vi "TCP Error Handler.vi"(3 "Error In":errorcluster, 4 "Info":string) -> (0 "Error Out":errorcluster, 1 "Info":string, 2 "TCP":bool)   [LabVIEW 2018]
doc: "Also checks for R&D FW or DAS FW"
uses:
  Type Defs/RT Command.ctl
  Type Defs/Global Action.ctl
  GC-MSMSDevlopment/Configuration/_Global Configuration.vi
  <vilib>/Utility/error.llb/Error Cluster From Error Code.vi
  <vilib>/ErrorRing/Error Ring.xnode
panel:
  # "All TCP/IP Errors are handle by this methode"
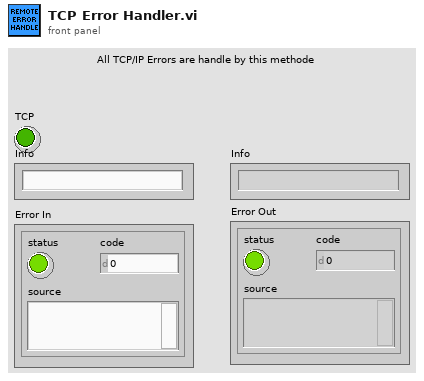
[diagram p1: front panel]
types:
  T1 = typedef "RT Command.ctl" = enum16{"xml Start Run", "xml Start Actual Run", "xml Stop Run", "xml Runtime Update", "xml Get Status", "xml Get Table", "xml Set Table", "xml Get Configuration", "xml System Status", "xml Set LC Input Logic", "xml Get Data", "xml Get Info", "Start", "StartActualRun", "Stop", "Runtime Update", "Get Data", "Get Info", "Get Status", "Get Param", "Get Config", "Get Table", "Read ADC", "Set Oscillator", "Update Config", "Update Table", "Set All Pol", "Set Pol and DC", "Set Max Mass", "Toggle RP", "Toggle EL", "Set PIC", "Initialize Turbo", "Send Turbo Comm", "Close Turbo", "P1", "P2", "P3", "Send Serial", "Set LC Out", "Get LC In", "Read VAC", "Test Table", "Toggle Power", "Get Startup", "Set Startup", "Get ADC Table", "Set ADC Table", "Get Brief Status", "Get Detail Status", "Auxiliary Update", "Set CC Logics", "Set CC Input Logics", "Ignore Error", "invalid"}
  T2 = typedef "Global Action.ctl" = enum16{"Write", "Read"}
  T3 = typedef "Global Configrations.ctl" = cluster{"Model Name":enum16{"QSight 110", "QSight 120", "QSight 210", "QSight 220", "QSight 410", "QSight 420", "IONICS 3Q 110", "IONICS 3Q 120", "IONICS 3Q 210", "IONICS 3Q 220", "IONICS 3Q 310", "IONICS 3Q 320", "Simulation (Single Source)", "Simulation (Dual Source)"}, "RunType":u16, "Acquisition State":enum16{"Ready", "Busy", "Waiting"}, "InstrState":enum16{"Initializing", "Mass Spectrometer is Off", "Starting Up", "Turning Power Off", "Going to Standby", "Roughing Pump Ready", "Turning Turbo Off", "Turbo Startup", "Turbopump Ready", "Checking Vacuum", "Going to Ready", "Ready", "Running", "Source Standby", "Lost Communication", "Shutting Down", "Fault", "24V Standby", "Go to 24V Standby", "Turbopump Ready-Waiting"}, "Run Mode":enum16{"MRM (Q1/Q2)", "Q1 Scan", "Q1 SRM", "Q2 Scan", "Q2 SRM", "Product Scan", "Precursor Scan", "Neutral Loss", "Neutral Gain"}, "Configration":T4, "TCP ID":refnum<k5>, "DT":bool, "Dead Time (nS)":i32, "Single Source":bool}
  T4 = typedef "Configration.ctl" = cluster{"Table":T5[], "Instrument":string[]}
  T5 = typedef "_RT Configuration 2.ctl" = cluster{"Name":string, "Ch#":u8, "Min":dbl, "Max":dbl, "Def+":dbl, "Def-":dbl, "Offset":dbl, "Slope":dbl, "Type":u8, "Description":string, "SettleT":dbl}
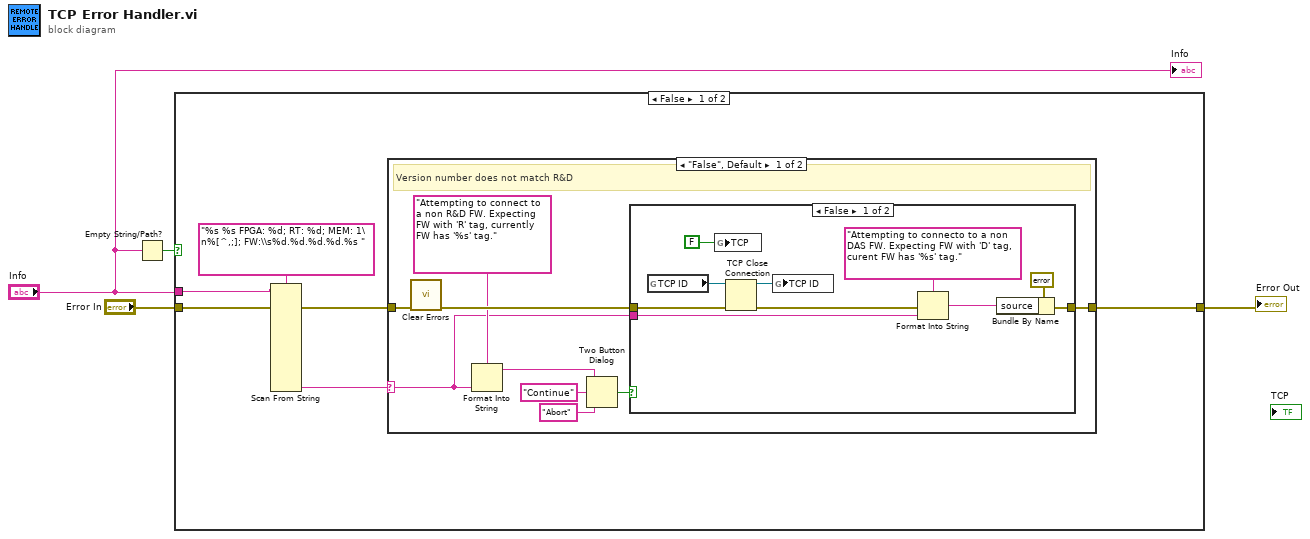
[diagram p0: block diagram]
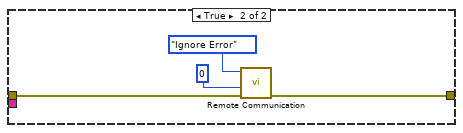
[diagram p2: hidden frame]
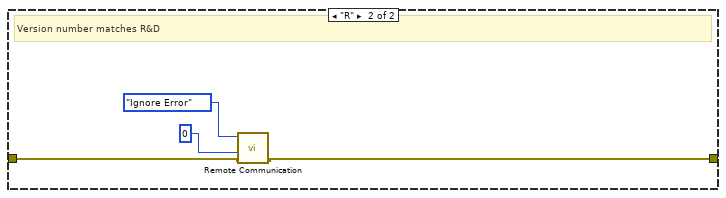
[diagram p3: hidden frame]
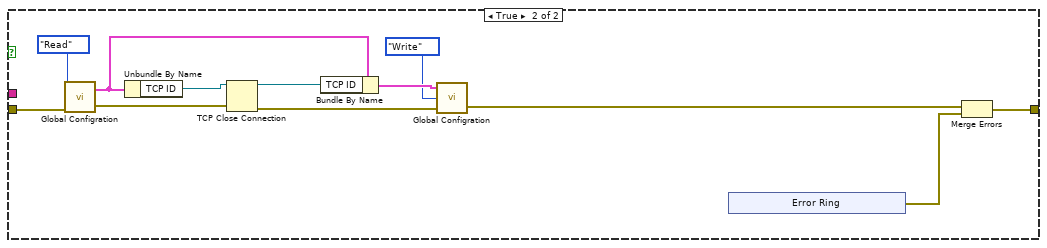
[diagram p4: hidden frame]
diagram:
  n1 = Empty String/Path?(string/path="Info") -> (empty?=w2:bool)
  n2 = case shown="False" w2 {
    tunnel: "Error In" -> [w8 w49]
    tunnel: [w10 w43] -> w4
    tunnel: "Info" -> [w5 _]
    frame False {
      n3 = Scan From String(format string="%s %s FPGA: %d; RT: %d; MEM: 1\n%[^,;]; FW:\\s%d.%d.%d.%d.%s ", input string=w5, error in=w8) -> (error out=w7:errorcluster, output 10=w6:string)  [unwired: 20 in, 2 out]
      n4 = case shown="\"False\", Default" w6 {
        selector: w6 -> [w11 _]
        tunnel: [w14 w37] -> w10
        tunnel: w7 -> [w19 w36]
        frame "False", Default {
          # "Version number does not match R&D"
          n5 = call <vilib>:"Clear Errors.vi"("error in (no error)"=w19) -> ("error out"=w15:errorcluster)  [unwired: 5 in, 1 out]
          n6 = Format Into String(format string="Attempting to connect to a non R&D FW. Expecting FW with 'R' tag, currently FW has '%s' tag." ("message"), w11) -> (resulting string=w12:string)  [unwired: 2 in, 1 out]
          n7 = Two Button Dialog(message=w12, 1:"Abort" ("F button name (\"Cancel\")"), 2:"Continue" ("T button name (\"OK\")")) -> (T button?=w16:bool)
          n8 = case shown="False" w16 {
            tunnel: w15 -> [w27 w32]
            tunnel: [w21 w33] -> w14
            tunnel: w11 -> [w23 _]
            frame False {
              n9 = global read "_Global Configuration.vi" "TCP ID"() -> (w29:refnum<k5>)
              n10 = global write "_Global Configuration.vi" "TCP"(FALSE) -> ()
              n11 = TCP Close Connection(connection ID=w29, error in (no error)=w27) -> (connection ID out=w28:refnum<k5>, error out=w22:errorcluster)  [unwired: 1 in]
              n12 = global write "_Global Configuration.vi" "TCP ID"(w28) -> ()
              n13 = Format Into String(format string="Attempting to connecto to a non DAS FW. Expecting FW with 'D' tag, curent FW has '%s' tag." ("source"), error in=w22, w23) -> (resulting string=w24:string)  [unwired: 1 in, 1 out]
              n14 = Bundle By Name(cluster=errorcluster {"status"=TRUE, "code"=110, "source"="Attempting to connecto to a non MD FW"} ("error out"), "source"=w24) -> (w21:errorcluster)
            }
            frame True {
              n15 = call "Remote Communication.vi"("Error In"=w32, "DC Param"=u16 0, "Command"=RT_Command."Ignore Error") -> ("Error Out"=w33:errorcluster)  [unwired: 3 in, 3 out]
            }
          }
        }
        frame "R" {
          # "Version number matches R&D"
          n16 = call "Remote Communication.vi"("Error In"=w36, "DC Param"=u16 0, "Command"=RT_Command."Ignore Error") -> ("Error Out"=w37:errorcluster)  [unwired: 3 in, 3 out]
        }
      }
    }
    frame True {
      n17 = call "Global Configration.vi"("Error In"=w49, "Action"=Global_Action."Read") -> ("Error Out"=w48:errorcluster, "Parameters Out"=w38:T3)  [unwired: 1 in]
      n18 = Unbundle By Name(w38) -> ("TCP ID"=w47:refnum<k5>)
      n19 = TCP Close Connection(connection ID=w47, error in (no error)=w48) -> (connection ID out=w44:refnum<k5>, error out=w46:errorcluster)  [unwired: 1 in]
      n20 = Bundle By Name(cluster=w38, "TCP ID"=w44) -> (w45:T3)
      n21 = call "Global Configration.vi"("Error In"=w46, "Action"=Global_Action."Write", "Parameters In"=w45) -> ("Error Out"=w41:errorcluster)  [unwired: 1 out]
      n22 = xnode "Error Ring"() -> ("error out"=w42:errorcluster)
      n23 = Merge Errors(w41, w42) -> (w43:errorcluster)
    }
  }
  "Error Out" <- w4
  "Info" <- "Info"
